vi "Catapult GetSet.vi"(9 "Enum":enum16{"Set", "Get"}(ring), 10 "CatapultDevRef in":T1={"Catapult State Reference"=refnum, "SolenoidDevRef"={"DevStatus"={"status"=FALSE, "code"=0, "source"=""}, "Pneumatics Control Module"=0, "Forward Solenoid Channel"=enum."Invalid", "Reverse Solenoid Channel"=enum."Invalid"}, "Catapult Configuration Reference"=refnum}, 11 "DevRef":string) -> (0 "Error Out":errorcluster, 3 "CatapulDevRef out":T1={"Catapult State Reference"=refnum, "SolenoidDevRef"={"DevStatus"={"status"=FALSE, "code"=0, "source"=""}, "Pneumatics Control Module"=0, "Forward Solenoid Channel"=enum."Invalid", "Reverse Solenoid Channel"=enum."Invalid"}, "Catapult Configuration Reference"=refnum})   [LabVIEW 2015]
uses:
  <userlib>/836 Library/Pneumatics/Catapult/836_CatapultDevRef.ctl
  <userlib>/836 Library/Pneumatics/Catapult/Catapult State.ctl
  <userlib>/836 Library/Pneumatics/Catapult/CatapultStateMachine.ctl
  <userlib>/836 Library/Pneumatics/Catapult/836_CatapultActions.ctl
  <vilib>/Rock Robotics/WPI/Solenoid/WPI_SolenoidDevRef.ctl
  <vilib>/Rock Robotics/WPI/Solenoid/WPI_SolenoidChannel.ctl
  <userlib>/836 Library/Pneumatics/Catapult/Catapult Configuration.ctl
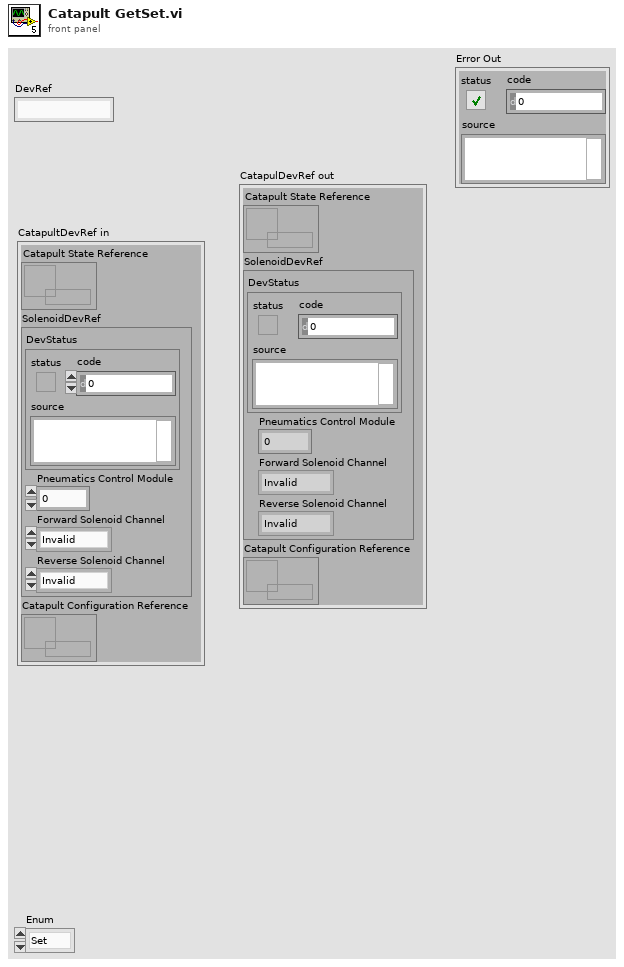
[diagram p1: front panel]
types:
  T1 = typedef "836_CatapultDevRef.ctl" = cluster{"Catapult State Reference":refnum<data-value>, "SolenoidDevRef":T2, "Catapult Configuration Reference":refnum<data-value>}
  T2 = typedef "WPI_SolenoidDevRef.ctl" = cluster{"DevStatus":errorcluster, "Pneumatics Control Module":u8, "Forward Solenoid Channel":T3, "Reverse Solenoid Channel":T3}
  T3 = typedef "WPI_SolenoidChannel.ctl" = enum8{"Solenoid 0", "Solenoid 1", "Solenoid 2", "Solenoid 3", "Solenoid 4", "Solenoid 5", "Solenoid 6", "Solenoid 7", "Invalid"}
  T4 = typedef "Catapult State.ctl" = cluster{"Position":bool, "Initialize":bool, "First Action?":bool, "Current State":T5, "Multiuse Timer":u32, "Second Action":T6}
  T5 = typedef "CatapultStateMachine.ctl" = enum8{"Status", "Forward", "Back", "Timed Forward", "Timed Back", "Analog Forwad", "Analog Back", "Digital Forward", "Digital Back", "Off"}
  T6 = typedef "836_CatapultActions.ctl" = enum8{"Fire", "Fire Timed", "Fire Analog", "Fire Digital", "Retract", "Retract Timed", "Retract Analog", "Retract Digital", "Hold", "Toggle", "Toggle Timed", "Toggle Analog", "Toggle Digital"}
  T7 = typedef "Catapult Configuration.ctl" = cluster{"Time Forward":u32, "Time Back":u32, "Digital Forward Samples":u32, "Digital Backward Samples":u32, "Analog Forward Settling Time":u32, "Analog Backward Settling Time":u32, "Analog Forward Threshold":sgl, "Analog Backward Threshold":sgl}
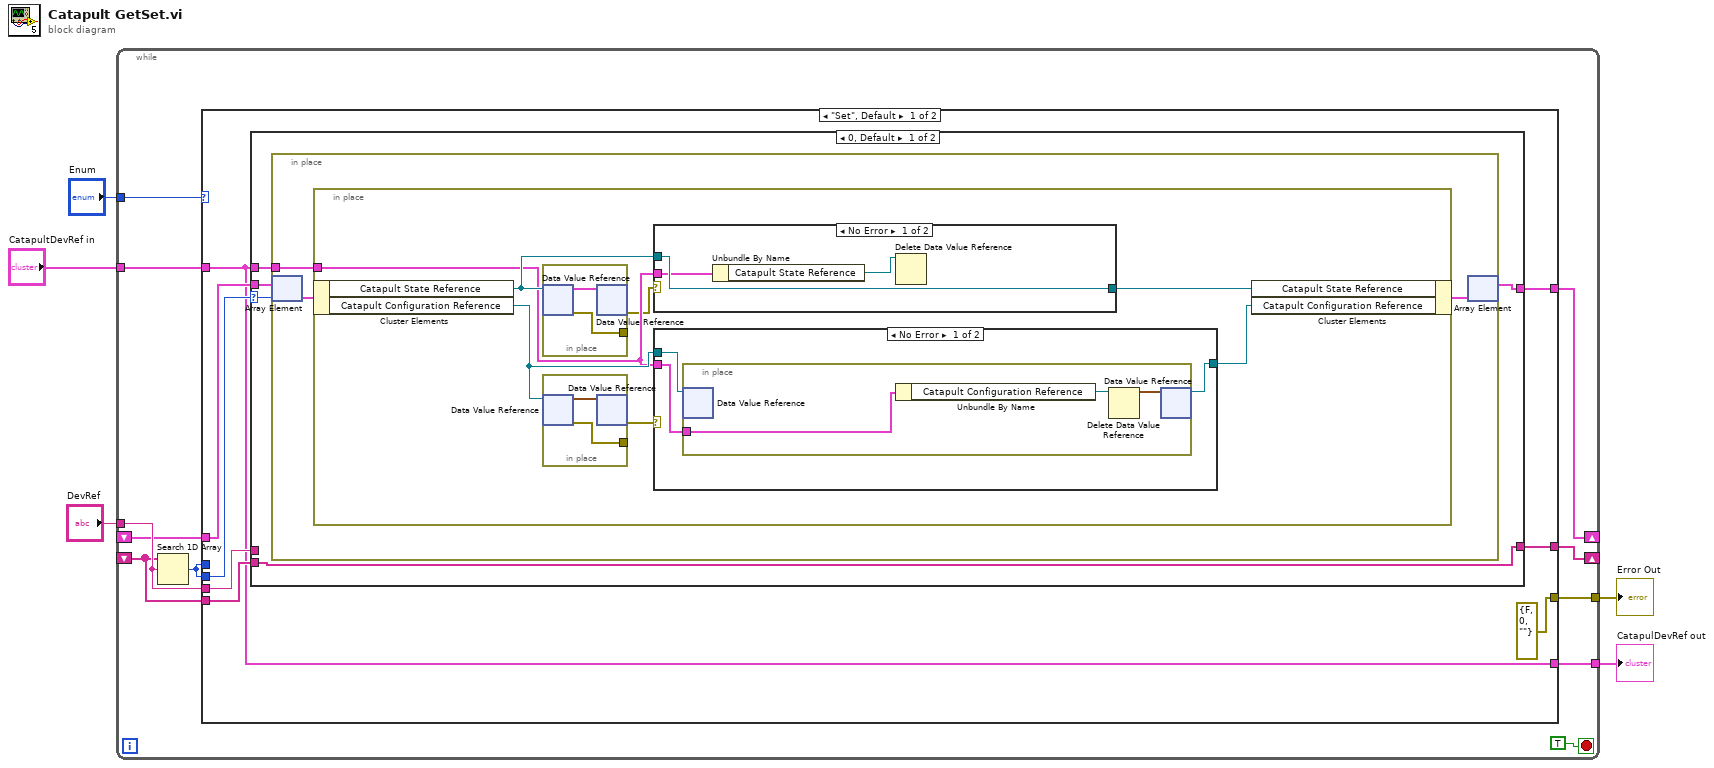
[diagram p0: block diagram]
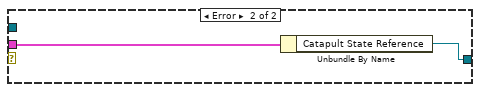
[diagram p2: hidden frame]
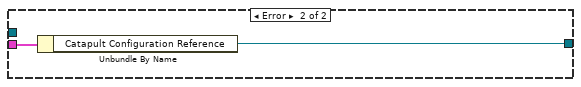
[diagram p3: hidden frame]
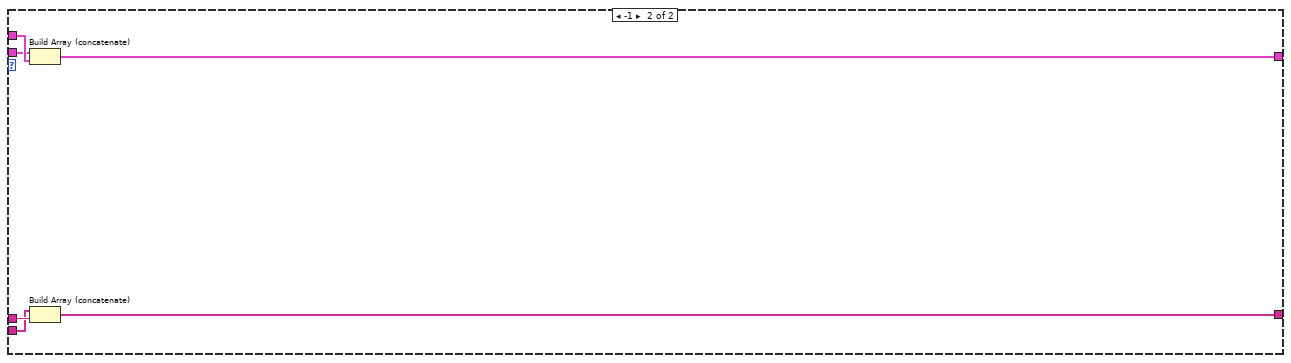
[diagram p4: hidden frame]
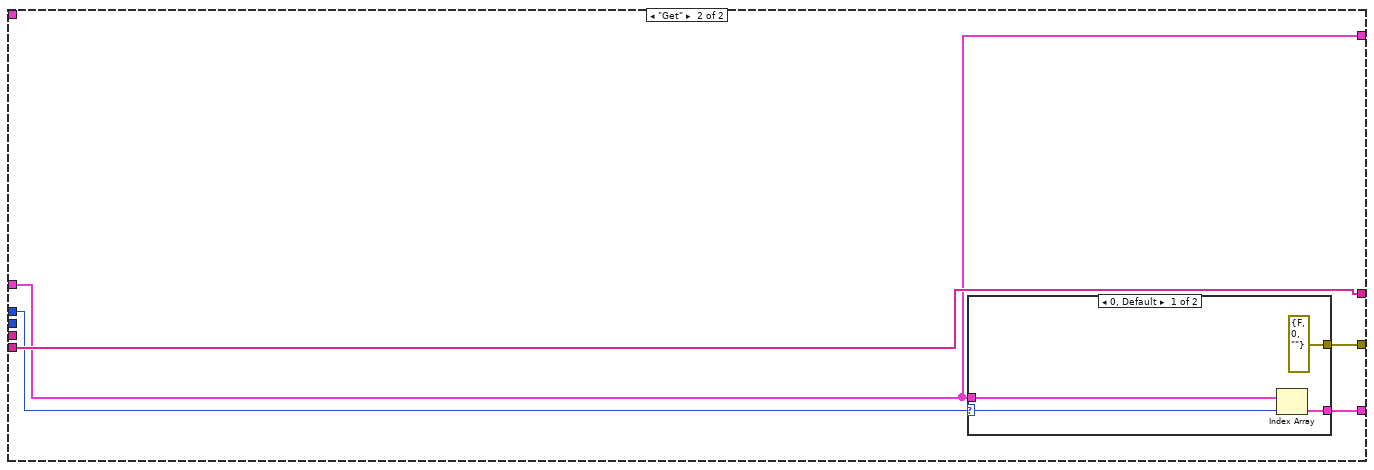
[diagram p5: hidden frame]
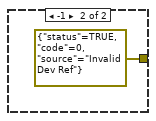
[diagram p6: hidden frame]
diagram:
  n1 = while {
    shift-right: [w12] -> _
    shift-left: _ -> [w11]
    shift-right: [w15] -> _
    shift-left: _ -> [w14]
    tunnel: "DevRef" -> [w16]
    tunnel: "CatapultDevRef in" -> [w13]
    tunnel: [w8] -> w4
    tunnel: "Enum" -> [w7]
    tunnel: [w6] -> w1
    stop <- TRUE stop-if-true
    n2 = Search 1D Array(1D array=w14, element=w16) -> (index of element=w9:i32)  [unwired: 1 out]
    n3 = case shown="\"Set\", Default" w7 {
      tunnel: w9 -> [w24 _]
      tunnel: w16 -> [w23 _]
      tunnel: [w22 w67] -> w15
      tunnel: w14 -> [w21 w67]
      tunnel: w13 -> [w18 _]
      tunnel: [w20 w66] -> w12
      tunnel: w11 -> [w19 w66]
      tunnel: w9 -> [_ w65]
      tunnel: [w18 w64] -> w8
      tunnel: [errorcluster {"status"=FALSE, "code"=0, "source"=""} ("error constant") w63] -> w6
      frame "Set", Default {
        n4 = case shown="0, Default" w24 {
          selector: w24 -> [w29 _]
          tunnel: [w25 w62] -> w20
          tunnel: [w28 w61] -> w22
          tunnel: w23 -> [_ w60]
          tunnel: w21 -> [w28 w59]
          tunnel: w18 -> [w26 w58]
          tunnel: w19 -> [w27 w57]
          frame 0, Default {
            n5 = in-place {
              in-place-border: w26 -> [w30]
              n6 = in-place-array #1(w27, w29) -> (w32:T1)
              n7 = in-place {
                in-place-border: w30 -> [w35]
                n8 = in-place-cluster #2(w32) -> ("Catapult State Reference"=w36:refnum<data-value>, "Catapult Configuration Reference"=w38:refnum<data-value>)
                n9 = in-place {
                  in-place-border: [w46] -> _
                  n10 = in-place-dvr #3(w36) -> (w45:T4, w46:errorcluster)
                  n11 = in-place-dvr #3(w45) -> (w34:errorcluster)  [unwired: 1 out]
                }
                n12 = in-place {
                  in-place-border: [w56] -> _
                  n13 = in-place-dvr #4(w38) -> (w55:T7, w56:errorcluster)
                  n14 = in-place-dvr #4(w55) -> (w33:errorcluster)  [unwired: 1 out]
                }
                n15 = case shown="No Error" w34 {
                  tunnel: [w42 w43] -> w37
                  tunnel: w36 -> [w42 _]
                  tunnel: w35 -> [w41 w44]
                  frame No Error {
                    n16 = Unbundle By Name(w41) -> ("Catapult State Reference"=w40:refnum<data-value>)
                    n17 = Delete Data Value Reference(data value reference=w40) -> ()  [unwired: 1 in, 2 out]
                  }
                  frame Error {
                    n18 = Unbundle By Name(w44) -> ("Catapult State Reference"=w43:refnum<data-value>)
                  }
                }
                n19 = case shown="No Error" w33 {
                  tunnel: [w49 w53] -> w39
                  tunnel: w35 -> [w48 w54]
                  tunnel: w38 -> [w47 _]
                  frame No Error {
                    n20 = in-place {
                      in-place-border: w48 -> [w52]
                      n21 = in-place-dvr #5(w47) -> ()  [unwired: 2 out]
                      n22 = Unbundle By Name(w52) -> ("Catapult Configuration Reference"=w51:refnum<data-value>)
                      n23 = Delete Data Value Reference(data value reference=w51) -> (data value=w50:T7)  [unwired: 1 in, 1 out]
                      n24 = in-place-dvr #5(w50) -> (w49:refnum<data-value>)  [unwired: 1 out]
                    }
                  }
                  frame Error {
                    n25 = Unbundle By Name(w54) -> ("Catapult Configuration Reference"=w53:refnum<data-value>)
                  }
                }
                n26 = in-place-cluster #2("Catapult State Reference"=w37, "Catapult Configuration Reference"=w39) -> (w31:T1)
              }
              n27 = in-place-array #1(w31) -> (w25:T1[])  [unwired: 1 out]
            }
          }
          frame -1 {
            n28 = Build Array (concatenate)(w57, w58) -> (w62:T1[])
            n29 = Build Array (concatenate)(w59, w60) -> (w61:string[])
          }
        }
      }
      frame "Get" {
        n30 = case shown="0, Default" w65 {
          selector: w65 -> [w70 _]
          tunnel: w66 -> [w71 _]
          tunnel: [w69 _] -> w64
          tunnel: [errorcluster {"status"=FALSE, "code"=0, "source"=""} ("error constant") errorcluster {"status"=TRUE, "code"=0, "source"="Invalid Dev Ref"} ("error constant")] -> w63
          frame 0, Default {
            n31 = Index Array(array=w71, index=w70) -> (element=w69:T1)
          }
          frame -1 {
          }
        }
      }
    }
  }
  "CatapulDevRef out" <- w4
  "Error Out" <- w1
